vi "Element Type.vi"(11 "GaugeIndicator in":refnum<class "GaugeIndicator.lvclass">) -> (2 "Element Type":string)   [LabVIEW 2020, in "VolatusGUIElements.lvlib" / "GaugeIndicator.lvclass"]
uses:
  GaugeIndicator.lvclass
  GaugeIndicator.lvclass/GaugeIndicator.ctl
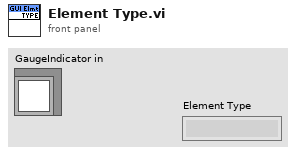
[diagram p1: front panel]
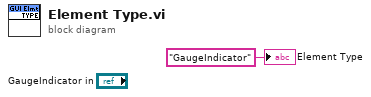
[diagram p0: block diagram]
diagram:
  "Element Type" <- "GaugeIndicator" ("Element Type")
